vi "ArmExecute.vi"(8 "error in (no error)":errorcluster) -> (0 "error out":errorcluster)   [LabVIEW 2023]
doc: "Arm Execute for 2024 robot"
uses:
  <vilib>/Rock Robotics/WPI/ThirdParty/JAS_Junk/TrajLib/Trajectory_Library.lvlib
  ArmGetSetpointEnum.ctl
  ArmNetworkingGlobal.vi
  ArmGlobal.vi
  <vilib>/Rock Robotics/WPI/ThirdParty/REV Robotics/REVLib/SubVI/Public/SPARK Get Encoder Status Position.vi
  <vilib>/Rock Robotics/WPI/ThirdParty/REV Robotics/REVLib/Typedef/Spark MAX Control Type.ctl
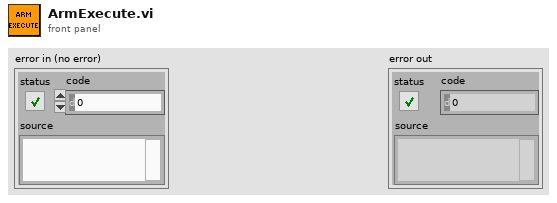
[diagram p1: front panel]
types:
  T1 = typedef "Spark MAX Control Type.ctl" = enum16{"Percent VBus", "Voltage", "Velocity", "Position", "Smart Motion", "Current", "Smart Velocity", "MAXMotion Position", "MAXMotion Velocity"}
  T2 = typedef "WPI_SwitchDevRef.ctl" = cluster{"DevStatus":errorcluster, "DIO Channel":T3, "CntIndex":T4, "Normally Closed":bool}
  T3 = typedef "FPGA_DIOChannel.ctl" = enum8{"DIO 0", "DIO 1", "DIO 2", "DIO 3", "DIO 4", "DIO 5", "DIO 6", "DIO 7", "DIO 8", "DIO 9", "DIO MXP 0", "DIO MXP 1", "DIO MXP 2", "DIO MXP 3", "DIO MXP 4", "DIO MXP 5", "DIO MXP 6", "DIO MXP 7", "DIO MXP 8", "DIO MXP 9", "DIO MXP 10", "DIO MXP 11", "DIO MXP 12", "DIO MXP 13", "DIO MXP 14", "DIO MXP 15", "SPI Port CS1", "SPI Port CS2", "SPI Port CS3", "SPI Port MISO", "SPI Port MOSI", "Invalid"}
  T4 = typedef "FPGA_CounterCtrSystemIndex.ctl" = enum8{"Ctr 0", "Ctr 1", "Ctr 2", "Ctr 3", "Ctr 4", "Ctr 5", "Ctr 6", "Ctr 7", "Invalid"}
  T5 = typedef "WPI_MotorControlDeviceRef.ctl" = cluster{"DeviceStatus":errorcluster, "Type":T6, "PWM":cluster{"PWM Channel":T7, "DeadBand":T8}, "CAN":cluster{"Device Number":u8, "SetOutput VI Ref":variant, "GetOutput VI Ref":variant, "Enable VI Ref":variant, "Disable VI Ref":variant, "Data":variant}, "Invert":bool, "DIO PWM":cluster{"PWM \"Enable\" Channel":T7, "DIOChannel":T3, "PWM Rate":dbl}}
  T6 = typedef "WPI_MotorControlType.ctl" = enum16{"PWM", "CAN", "DIO PWM"}
  T7 = typedef "FPGA_DIOPWMChannel.ctl" = enum8{"PWM 0", "PWM 1", "PWM 2", "PWM 3", "PWM 4", "PWM 5", "PWM 6", "PWM 7", "PWM 8", "PWM 9", "PWM MXP 0", "PWM MXP 1", "PWM MXP 2", "PWM MXP 3", "PWM MXP 4", "PWM MXP 5", "PWM MXP 6", "PWM MXP 7", "PWM MXP 8", "PWM MXP 9", "Invalid"}
  T8 = typedef "WPI_PWMDeadband.ctl" = cluster{"Name":string, "maxPositivePwm":i32, "minPositivePwm":i32, "centerPwm":i32, "maxNegativePwm":i32, "minNegativePwm":i32, "angularRange":u16}
  T9 = typedef "ArmGetSetpointEnum.ctl" = enum16{"ArmFloorPickup", "ArmAmpDeposit", "ArmSpeakerShoot", "ArmStartPosition", "ArmRestPosition", "ArmSourceIntake", "ArmAwayShoot"}
  T10 = typedef "Trajectory_Library.lvlib/PosCtrl_Tuning_Type.ctl" = cluster{"Slope":dbl, "Offset":dbl, "Error Deadband":dbl, "At Reference Count":i32, "Negate Output":bool, "Max Allowd Position":dbl, "Min Allowd Position":dbl}
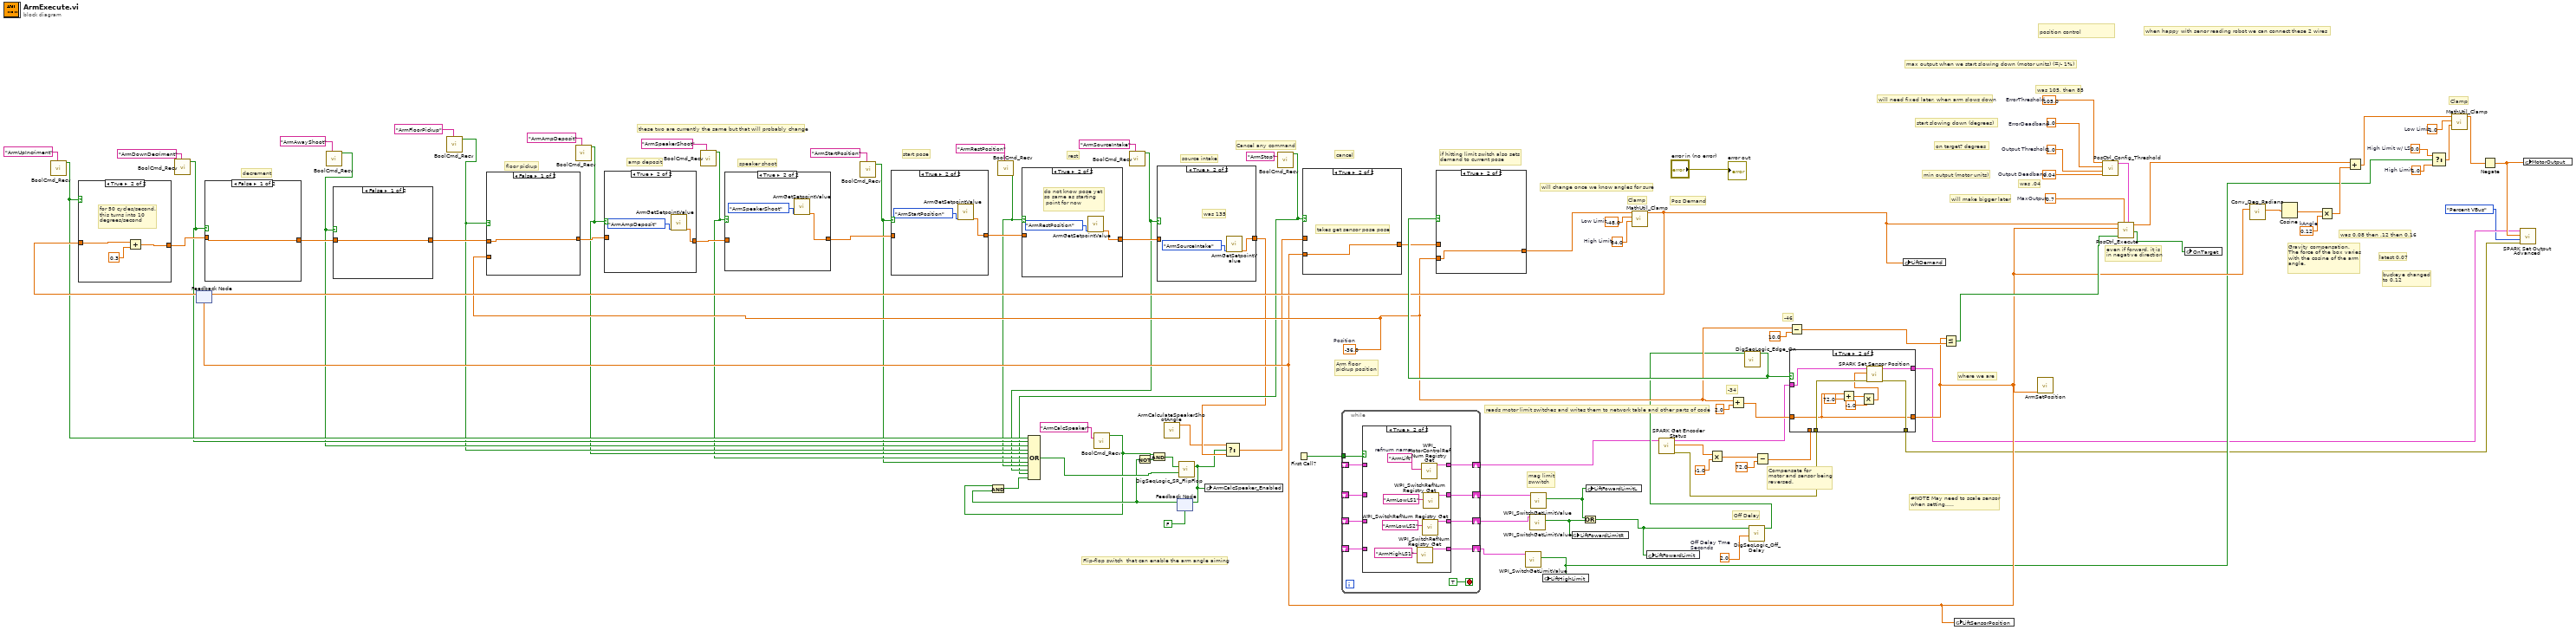
[diagram p0: block diagram]
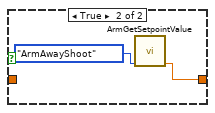
[diagram p3: hidden frame]
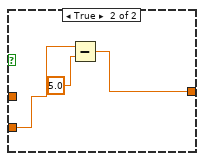
[diagram p11: hidden frame]
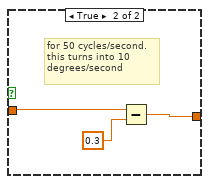
[diagram p12: hidden frame]
diagram:
  w10 = 0.0  # High Limit w/ LS
  w19 = 84.0  # High Limit
  w44 = 2.0  # Off Delay Tme Seconds
  w11 = 1.0  # High Limit
  w53 = -1.0  # Low Limit
  w47 = -36.0  # Position
  w69 = 0.12  # kAngle
  w86 = -48.0  # Low Limit
  w95 = 0.7  # MaxOutput
  w93 = 105.0  # ErrorThreshold
  w92 = 1.0  # ErrorDeadband
  w91 = 1.0  # Output Threshold
  w90 = 0.04  # Output Deadband
  # "buckeye changed\nto 0.12"
  # "latest 0.07"
  # "Flip-flop switch  that can enable the arm angle aiming"
  # "#NOTE May need to scale sensor \nwhen setting....."
  # "Off Delay"
  # "mag limit\nswwitch"
  # "-34"
  # "-46"
  # "Pos Demand"
  # "Clamp"
  # "was 105, then 85"
  # "was .04"
  # "was 0.08 then .12 then 0.16"
  # "Arm floor\npickup position"
  # "Gravity compensation.\nThe force of the box varies\nwith the cosine of the arm\nangle."
  # "Compensate for\nmotor and sensor being\nreversed."
  # "even if forward, it is \nin negative direction"
  # "if hitting limit switch also sets \ndemand to current pose"
  # "these two are currently the same but that will probably change"
  # "Cancel any command"
  # "source intake"
  # "will change once we know angles for sure"
  # "cancel"
  # "rest"
  # "start pose"
  # "speaker shoot"
  # "Clamp"
  # "amp deposit"
  # "floor pickup"
  # "decrement"
  # "when happy with senor reading robot we can connect these 2 wires"
  # "min output (motor units)"
  # "max output when we start slowing down (motor units) (=/- 1%)"
  # "on target? degrees"
  # "start slowing down (degrees)"
  # "will make bigger later"
  # "where we are"
  # "position control"
  # "will need fixed later, when arm slows down"
  # "reads motor limit switches and writes them to network table and other parts of code"
  n1 = call <vilib>:"BoolCmd_Recv.vi"("Command Name"="ArmUpIncriment") -> ("New Request"=w38:bool)  [unwired: 9 in, 1 out]
  n2 = call <vilib>:"BoolCmd_Recv.vi"("Command Name"="ArmDownDecriment") -> ("New Request"=w37:bool)  [unwired: 9 in, 1 out]
  n3 = call <vilib>:"BoolCmd_Recv.vi"("Command Name"="ArmAwayShoot") -> ("New Request"=w36:bool)  [unwired: 9 in, 1 out]
  n4 = call <vilib>:"BoolCmd_Recv.vi"("Command Name"="ArmFloorPickup") -> ("New Request"=w35:bool)  [unwired: 9 in, 1 out]
  n5 = call <vilib>:"BoolCmd_Recv.vi"("Command Name"="ArmAmpDeposit") -> ("New Request"=w34:bool)  [unwired: 9 in, 1 out]
  n6 = call <vilib>:"BoolCmd_Recv.vi"("Command Name"="ArmSpeakerShoot") -> ("New Request"=w33:bool)  [unwired: 9 in, 1 out]
  n7 = call <vilib>:"BoolCmd_Recv.vi"("Command Name"="ArmStartPosition") -> ("New Request"=w32:bool)  [unwired: 9 in, 1 out]
  n8 = call <vilib>:"BoolCmd_Recv.vi"("Command Name"="ArmRestPosition") -> ("New Request"=w31:bool)  [unwired: 9 in, 1 out]
  n9 = call <vilib>:"BoolCmd_Recv.vi"("Command Name"="ArmCalcSpeaker") -> ("New Request"=w23:bool)  [unwired: 9 in, 1 out]
  n10 = call <vilib>:"BoolCmd_Recv.vi"("Command Name"="ArmSourceIntake") -> ("New Request"=w30:bool)  [unwired: 9 in, 1 out]
  n11 = call "ArmCalculateSpeakerShootAngle.vi"() -> ("ArmAngle (degrees)"=w26:dbl)  [unwired: 11 in]
  n12 = feedback #1(FALSE ("Output")) -> (w24:bool)
  n13 = And(x=w23, y=w24) -> (x .and. y?=w22:bool)
  n14 = Not(x=w24) -> (.not. x?=w40:bool)
  n15 = And(x=w23, y=w40) -> (x .and. y?=w39:bool)
  n16 = call <vilib>:"BoolCmd_Recv.vi"("Command Name"="ArmStop") -> ("New Request"=w29:bool)  [unwired: 9 in, 1 out]
  n17 = Compound Arithmetic op=OR(w38, w37, w36, w35, w34, w33, w32, w31, w30, w29, w22) -> (w25:bool)
  n18 = call <vilib>:"DigSeqLogic_SR_FlipFlop.vi"("Set"=w39, "Reset"=w25) -> ("Output"=w20:bool)  [unwired: 12 in, 1 out]
  n19 = feedback-in #1(w20) -> ()
  n20 = global write "ArmGlobal.vi" "ArmCalcSpeaker_Enabled"(w20) -> ()
  n21 = First Call?() -> (First Call?: T/F=w56:bool)
  n22 = while {
    tunnel: w56 -> [w104]
    shift-right: [w105] -> w8
    shift-left: _ -> [w102]
    shift-right: [w101] -> w54
    shift-left: _ -> [w100]
    shift-right: [w99] -> w18
    shift-left: _ -> [w98]
    shift-right: [w97] -> w14
    shift-left: _ -> [w96]
    stop <- TRUE stop-if-true
    n23 = case shown="True" w104 {
      tunnel: [w109 w117] -> w105
      tunnel: w102 -> [w109 _]
      tunnel: [w108 w114] -> w101
      tunnel: w100 -> [w108 _]
      tunnel: [w107 w112] -> w99
      tunnel: w98 -> [w107 _]
      tunnel: [w106 w110] -> w97
      tunnel: w96 -> [w106 _]
      frame False {
      }
      frame True {
        w116 = "ArmLift"  # refnum name
        n24 = call <vilib>:"WPI_SwitchRefNum Registry Get.vi"("refnum name"="ArmHighLS1") -> ("SwitchDevRef"=w110:T2)  [unwired: 9 in, 1 out]
        n25 = call <vilib>:"WPI_MotorControlRefNum Registry Get.vi"("refnum name"=w116) -> ("MotorControlDevRef"=w117:T5)  [unwired: 9 in, 1 out]
        n26 = call <vilib>:"WPI_SwitchRefNum Registry Get.vi"("refnum name"="ArmLowLS2") -> ("SwitchDevRef"=w112:T2)  [unwired: 9 in, 1 out]
        n27 = call <vilib>:"WPI_SwitchRefNum Registry Get.vi"("refnum name"="ArmLowLS1") -> ("SwitchDevRef"=w114:T2)  [unwired: 9 in, 1 out]
      }
    }
  }
  n28 = call <vilib>:"WPI_SwitchGetLimitValue.vi"("SwitchDevRef"=w14) -> ("Switch Pressed"=w9:bool)  [unwired: 8 in, 2 out]
  n29 = call <vilib>:"WPI_SwitchGetLimitValue.vi"("SwitchDevRef"=w18) -> ("Switch Pressed"=w16:bool)  [unwired: 8 in, 2 out]
  n30 = call <vilib>:"WPI_SwitchGetLimitValue.vi"("SwitchDevRef"=w54) -> ("Switch Pressed"=w17:bool)  [unwired: 8 in, 2 out]
  n31 = global write "ArmNetworkingGlobal.vi" "LiftHighLimit"(w9) -> ()
  n32 = global write "ArmNetworkingGlobal.vi" "LiftFowardLimitR"(w16) -> ()
  n33 = Or(x=w17, y=w16) -> (x .or. y?=w15:bool)
  n34 = global write "ArmNetworkingGlobal.vi" "LiftFowardLimitL"(w17) -> ()
  n35 = global write "ArmNetworkingGlobal.vi" "LiftFowardLimit"(w15) -> ()
  n36 = call-poly <vilib>:"SPARK Get Encoder Status.vi"("MotorControlDevRef in"=w8) -> ("error out"=w7:errorcluster, "Sensor Position"=w6:dbl, "MotorControlDevRef out"=w5:T5)  [unwired: 7 in, 1 out]
  n37 = Multiply(x=w6, y=-1.0) -> (x*y=w65:dbl)
  n38 = Add(x=w47, y=2.0) -> (x+y=w50:dbl)
  n39 = call <vilib>:"DigSeqLogic_Off_Delay.vi"("Delay"=w44, "Input"=w15) -> ("Output"=w43:bool)  [unwired: 8 in, 1 out]
  n40 = call <vilib>:"DigSeqLogic_Edge_On.vi"("Input"=w43) -> ("On Edge"=w62:bool)  [unwired: 10 in]
  n41 = Subtract(x=w65, y=72.0) -> (x-y=w63:dbl)
  n42 = Subtract(x=w47, y=10.0) -> (x-y=w45:dbl)
  n43 = case shown="True" w62 {
    tunnel: [w119 w129] -> w2
    tunnel: [w120 w125] -> w42
    tunnel: w63 -> [w120 _]
    tunnel: w5 -> [w119 w128]
    tunnel: w50 -> [_ w125]
    tunnel: w7 -> [w118 w127]
    tunnel: [w118 w126] -> w3
    frame False {
    }
    frame True {
      n44 = Add(x=w125, y=72.0) -> (x+y=w124:dbl)
      n45 = Multiply(x=w124, y=-1.0) -> (x*y=w121:dbl)
      n46 = call <vilib>:"SPARK Set Sensor Position.vi"("error in"=w127, "Position"=w121, "MotorControlDeviceRef"=w128) -> ("error out"=w126:errorcluster, "MotorControlDeviceRef"=w129:T5)  [unwired: 7 in]
    }
  }
  n47 = feedback #2(w42) -> (w89:dbl)
  n48 = case shown="True" w38 {
    tunnel: w89 -> [w130 w133]
    tunnel: [w130 w131] -> w88
    frame False {
    }
    frame True {
      # "for 50 cycles/second.\nthis turns into 10 \ndegrees/second"
      n49 = Add(x=w133, y=0.3) -> (x+y=w131:dbl)
    }
  }
  n50 = case shown="False" w37 {
    tunnel: w88 -> [w134 w136]
    tunnel: [w134 w135] -> w59
    frame False {
    }
    frame True {
      # "for 50 cycles/second.\nthis turns into 10 \ndegrees/second"
      n51 = Subtract(x=w136, y=0.3) -> (x-y=w135:dbl)
    }
  }
  n52 = case shown="False" w36 {
    tunnel: w59 -> [w138 _]
    tunnel: [w138 w139] -> w58
    frame False {
    }
    frame True {
      n53 = call "ArmGetSetpointValue.vi"("ArmSetpoints"=ArmGetSetpointEnum."ArmAwayShoot") -> ("Setpoint"=w139:dbl)  [unwired: 10 in]
    }
  }
  n54 = case shown="False" w35 {
    tunnel: w58 -> [w141 _]
    tunnel: [w141 w143] -> w87
    tunnel: w47 -> [_ w144]
    frame False {
    }
    frame True {
      n55 = Subtract(x=w144, y=5.0) -> (x-y=w143:dbl)
    }
  }
  n56 = case shown="True" w34 {
    tunnel: w87 -> [w145 _]
    tunnel: [w145 w146] -> w85
    frame False {
    }
    frame True {
      n57 = call "ArmGetSetpointValue.vi"("ArmSetpoints"=ArmGetSetpointEnum."ArmAmpDeposit") -> ("Setpoint"=w146:dbl)  [unwired: 10 in]
    }
  }
  n58 = case shown="True" w33 {
    tunnel: w85 -> [w148 _]
    tunnel: [w148 w149] -> w84
    frame False {
    }
    frame True {
      n59 = call "ArmGetSetpointValue.vi"("ArmSetpoints"=ArmGetSetpointEnum."ArmSpeakerShoot") -> ("Setpoint"=w149:dbl)  [unwired: 10 in]
    }
  }
  n60 = case shown="True" w32 {
    tunnel: w84 -> [w151 _]
    tunnel: [w151 w152] -> w83
    frame False {
    }
    frame True {
      n61 = call "ArmGetSetpointValue.vi"("ArmSetpoints"=ArmGetSetpointEnum."ArmStartPosition") -> ("Setpoint"=w152:dbl)  [unwired: 10 in]
    }
  }
  n62 = case shown="True" w31 {
    tunnel: w83 -> [w154 _]
    tunnel: [w154 w155] -> w82
    frame False {
    }
    frame True {
      # "do not know pose yet \nso same as starting\n point for now"
      n63 = call "ArmGetSetpointValue.vi"("ArmSetpoints"=ArmGetSetpointEnum."ArmRestPosition") -> ("Setpoint"=w155:dbl)  [unwired: 10 in]
    }
  }
  n64 = case shown="True" w30 {
    tunnel: w82 -> [w157 _]
    tunnel: [w157 w158] -> w28
    frame False {
    }
    frame True {
      # "was 135"
      n65 = call "ArmGetSetpointValue.vi"("ArmSetpoints"=ArmGetSetpointEnum."ArmSourceIntake") -> ("Setpoint"=w158:dbl)  [unwired: 10 in]
    }
  }
  n66 = Select(t=w26, s=w20, f=w28) -> (s? t:f=w27:dbl)
  n67 = case shown="True" w29 {
    tunnel: w27 -> [w160 _]
    tunnel: [w160 w161] -> w60
    tunnel: w42 -> [_ w161]
    frame False {
    }
    frame True {
      # "takes get sensor pose pose"
    }
  }
  n68 = case shown="True" w62 {
    tunnel: w47 -> [_ w163]
    tunnel: [w162 w163] -> w61
    tunnel: w60 -> [w162 _]
    frame False {
    }
    frame True {
    }
  }
  n69 = call <vilib>:"MathUtil_Clamp.vi"("High Limit"=w19, "Low Limit"=w86, "Value"=w61) -> ("Result"=w51:dbl)  [unwired: 8 in]
  n70 = feedback-in #2(w51) -> ()
  n71 = global write "ArmNetworkingGlobal.vi" "LiftDemand"(w51) -> ()
  n72 = Less Or Equal?(x=w42, y=w45) -> (x <= y?=w48:bool)
  n73 = global write "ArmNetworkingGlobal.vi" "LiftSensorPosition"(w42) -> ()
  n74 = call "ArmSetPosition.vi"("ArmPos"=w42) -> ()  [unwired: 11 in]
  n75 = call <vilib>:"PosCtrl_Config_Threshold.vi"("Output Deadband"=w90, "Output Threshold"=w91, "ErrorDeadband"=w92, "ErrorThreshold"=w93) -> ("PosCtrl_Config_Params"=w94:T10)  [unwired: 7 in]
  n76 = call <vilib>:"PosCtrl_Execute.vi"("PosCtrl_Config_Params"=w94, "MaxOutput"=w95, "Rev Limit Switch"=w48, "CurrentPosition"=w42, "TargetPosition"=w51) -> ("OnTarget"=w55:bool, "Output"=w71:dbl)  [unwired: 4 in, 1 out]
  n77 = global write "ArmNetworkingGlobal.vi" "OnTarget"(w55) -> ()
  n78 = call <vilib>:"Conv_Deg_Radians.vi"("Degress"=w42) -> ("Radians"=w67:dbl)  [unwired: 10 in]
  n79 = Cosine(x=w67) -> (cos(x)=w68:dbl)
  n80 = Multiply(x=w68, y=w69) -> (x*y=w70:dbl)
  n81 = Add(x=w71, y=w70) -> (x+y=w13:dbl)
  n82 = Select(t=w10, s=w9, f=w11) -> (s? t:f=w12:dbl)
  n83 = call <vilib>:"MathUtil_Clamp.vi"("High Limit"=w12, "Low Limit"=w53, "Value"=w13) -> ("Result"=w52:dbl)  [unwired: 8 in]
  n84 = Negate(x=w52) -> (-x=w4:dbl)
  n85 = call <vilib>:"SPARK Set Output Advanced.vi"("error in (no error)"=w3, "Control Mode"=Spark_MAX_Control_Type."Percent VBus", "Setpoint"=w4, "MotorControlDevRef"=w2) -> ()  [unwired: 6 in, 2 out]
  n86 = global write "ArmNetworkingGlobal.vi" "MotorOutput"(w4) -> ()
  "error out" <- "error in (no error)"
